vi "ReadServo_Position.vi"() -> ()   [LabVIEW 2017]
uses:
  <vilib>/myRIO/Common/Instrument Driver Framework/myRIO v1.0/UART/vis/myRIO v1.0 Close UART.vi
  <vilib>/myRIO/Common/Instrument Driver Framework/Utilities/vis/FPGA Ref Manager.vi
  <vilib>/myRIO/Common/Instrument Driver Framework/myRIO v1.0/myRIO v1.0 Reset FPGA.vi
  <vilib>/myRIO/Common/Instrument Driver Framework/myRIO v1.0/IRQ/vis/myRIO v1.0 IRQ Info FGV.vi
  <vilib>/myRIO/Common/Instrument Driver Framework/myRIO v1.0/IRQ/vis/myRIO v1.0 Timer IRQ Info FGV.vi
  <vilib>/myRIO/Common/Instrument Driver Framework/myRIO v1.0/IRQ/vis/myRIO v1.0 ISR Agent.vi
  <vilib>/myRIO/Instrument Drivers/Utilities/Utilities.lvlib
panel:
  out "error out":errorcluster
  out "Servo Position":u8
  in  "Controller ID#  (I2C Address)":u8=2 min=1 max=4
  in  "Set Servo Position (0 - 180 degrees)":u8(slide)=90 scale=0.0..180.0
  in  "Select Channel 2":string(combo)="Servo 1"
  in  "stop":bool
  in  "Select Channel":string(combo)="Servo 1"
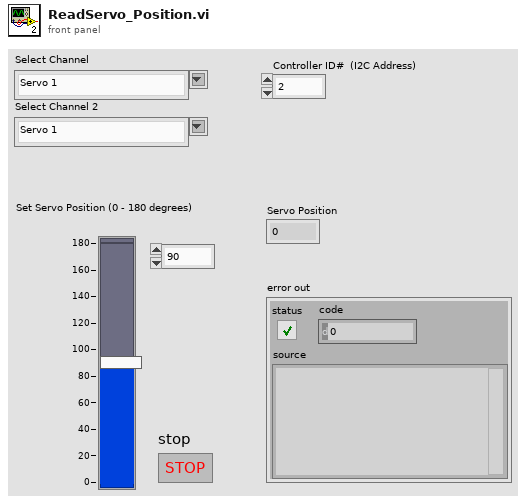
[diagram p1: front panel]
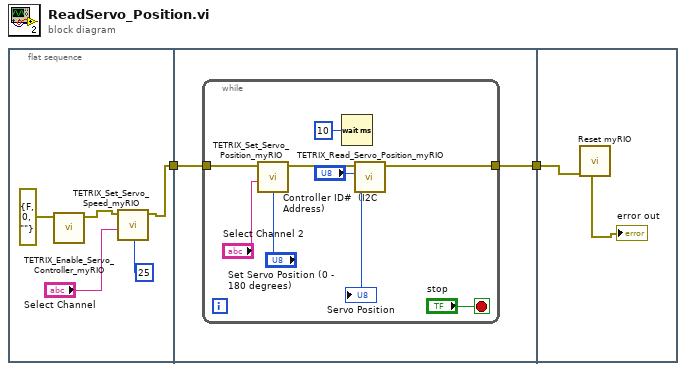
[diagram p0: block diagram]
diagram:
  n1 = flat-sequence {
    tunnel: [w3] -> w2
    tunnel: w2 -> [w9]
    tunnel: [w8] -> w1
    tunnel: w1 -> [w20]
    frame #0 {
      n2 = call <vilib>:"TETRIX_Enable_Servo_Controller_myRIO.vi"("Error/Flow In"=errorcluster {"status"=FALSE, "code"=0, "source"=""} ("error constant")) -> ("Error/Flow Out"=w6:errorcluster)  [unwired: 6 in]
      n3 = call <vilib>:"TETRIX_Set_Servo_Speed_myRIO.vi"("Set Servo Speed (0 - 100 percent)"=u8 25, "Select Channel"="Select Channel", "Error/Flow In"=w6) -> ("Error/Flow Out"=w3:errorcluster)  [unwired: 4 in]
    }
    frame #1 {
      n4 = while {
        tunnel: w9 -> [w16]
        tunnel: [w10] -> w8
        stop <- "stop" stop-if-true
        n5 = call <vilib>:"TETRIX_Set_Servo_Position_myRIO.vi"("Set Servo Position (0 - 180 degrees)"="Set Servo Position (0 - 180 degrees)", "Select Channel"="Select Channel 2", "Error/Flow In"=w16) -> ("Error/Flow Out"=w15:errorcluster)  [unwired: 4 in]
        n6 = Wait (ms)(milliseconds to wait=u32 10) -> ()  [unwired: 1 out]
        n7 = call <vilib>:"TETRIX_Read_Servo_Position_myRIO.vi"("Controller ID#  (I2C Address)"="Controller ID#  (I2C Address)", "Error/Flow In"=w15) -> ("Error/Flow Out"=w10:errorcluster, "Servo Position"=→"Servo Position":u8)  [unwired: 4 in]
      }
    }
    frame #2 {
      n8 = call <vilib>:"Reset myRIO.vi"("error in (no error)"=w20) -> ("error out"=→"error out":errorcluster)  [unwired: 10 in]
    }
  }
